vi "PD4-C Setup State Machine.vi"(11 "Boolean in":refnum<vi>) -> (0 "error out":errorcluster, 2 "Answer":i32, 3 "VISA Refnum out":refnum<visa-resource-name>)   [LabVIEW 2021]
uses:
  Nanotech PDC-4.lvlib
  <vilib>/Utility/error.llb/Error Cluster From Error Code.vi
  <vilib>/ErrorRing/Error Ring.xnode
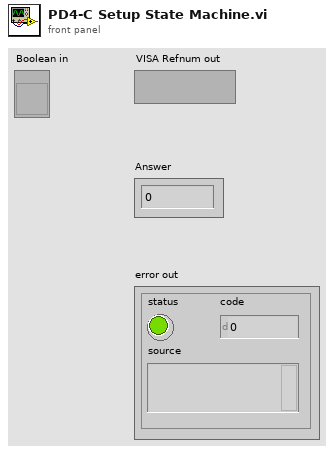
[diagram p1: front panel]
types:
  T1 = cluster{"Data (dec)":i32, "write":bool, "Index":string, "Sub-Index":string, "Data-Size (in Byte)":u8}
  T2 = cluster{"Index":string, "Sub-Index":string, "Data-Size (in Byte)":u8}
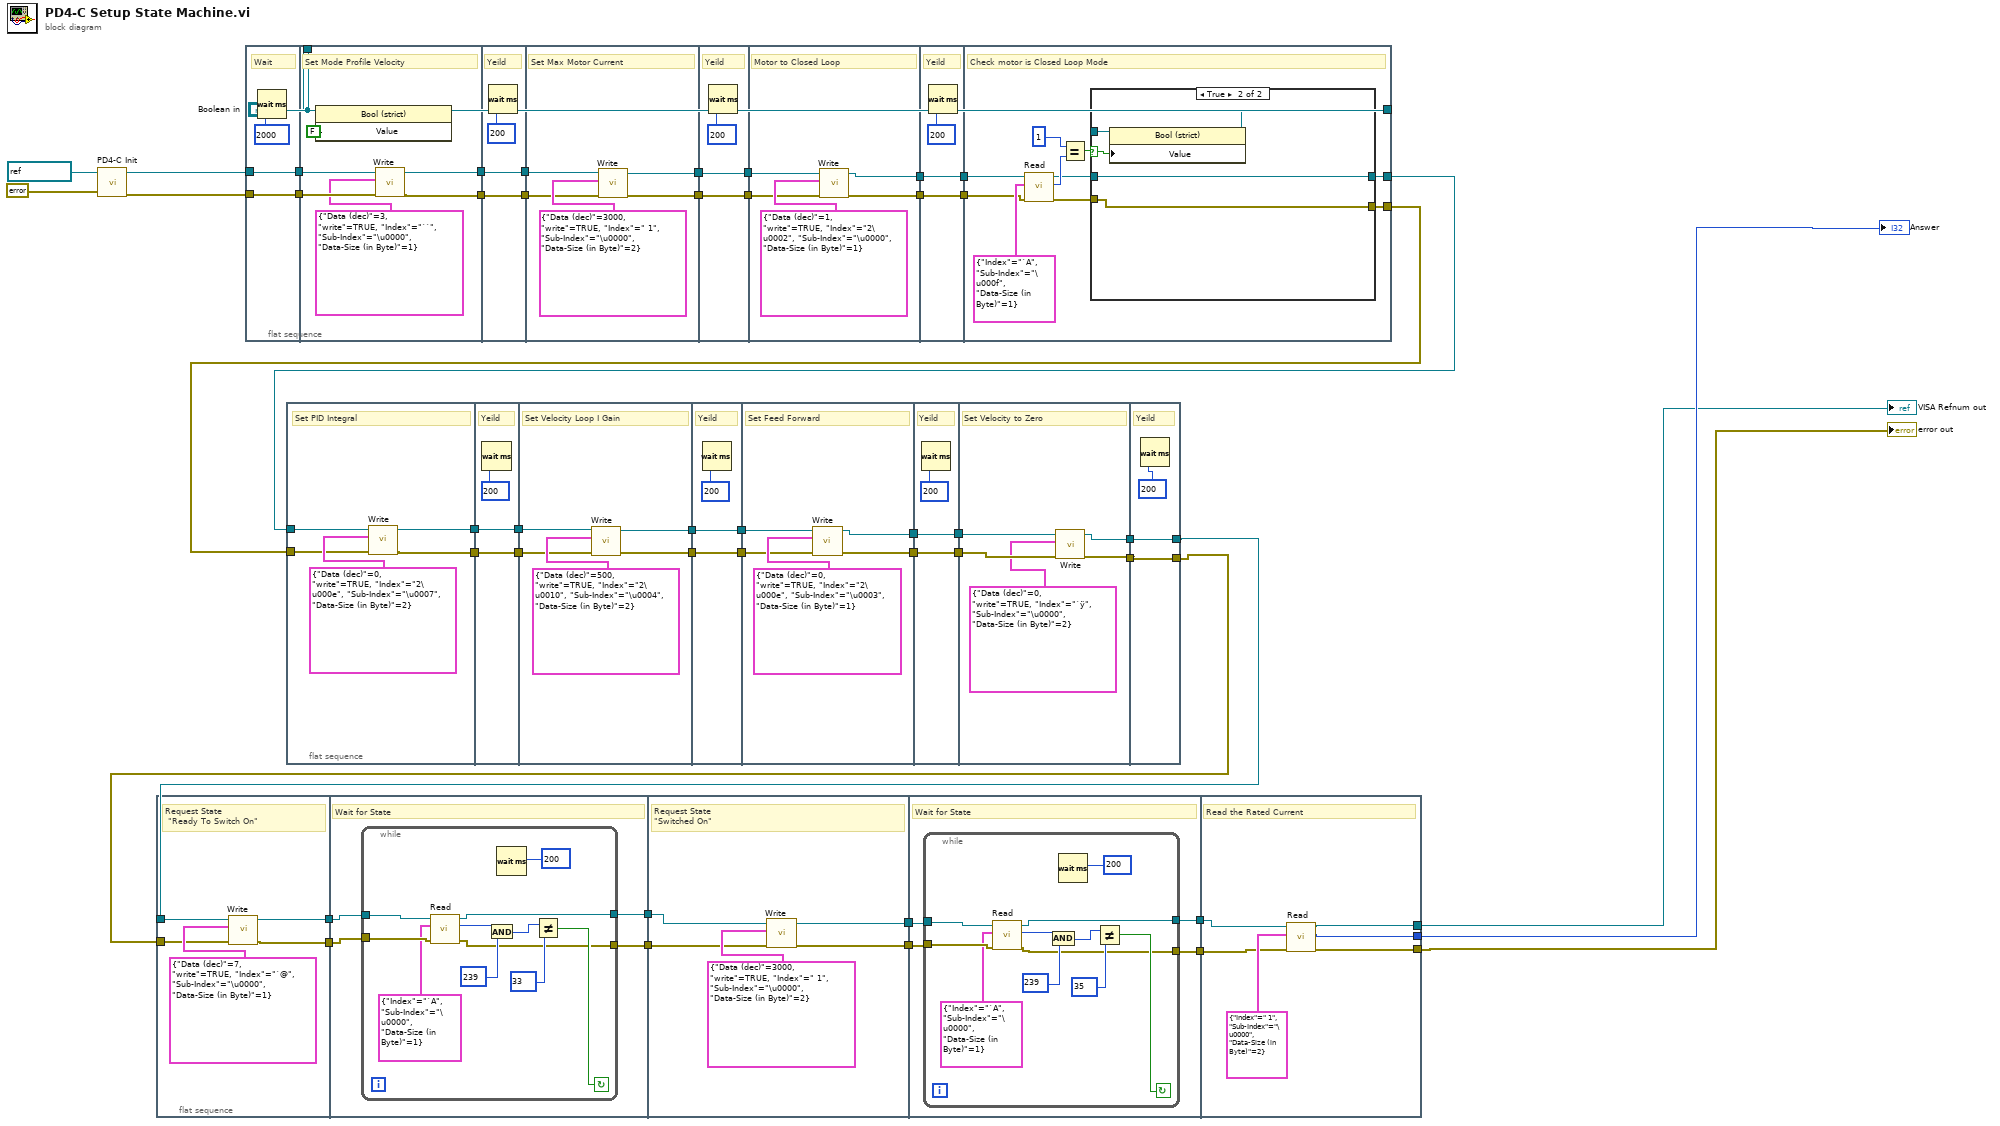
[diagram p0: block diagram]
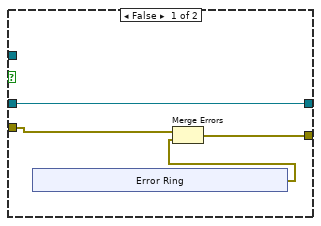
[diagram p2: hidden frame]
diagram:
  n1 = call "PD4-C Init.vi"("error in (no error)"=errorcluster {"status"=FALSE, "code"=0, "source"=""}, "VISA Refnum in"=refnum<visa-resource-name> "COM15") -> ("error out"=w4:errorcluster, "VISA Refnum out"=w5:refnum<visa-resource-name>)  [unwired: 8 in]
  n2 = flat-sequence {
    tunnel: [w52] -> w20
    tunnel: [w51] -> w19
    tunnel: w8 -> [w50]
    tunnel: w9 -> [w49]
    tunnel: w20 -> [w56]
    tunnel: w19 -> [w57]
    tunnel: [w55] -> w18
    tunnel: [w54] -> w17
    tunnel: [w72] -> w16
    tunnel: [w71] -> w15
    tunnel: w18 -> [w70]
    tunnel: w17 -> [w69]
    tunnel: w16 -> [w76]
    tunnel: w15 -> [w77]
    tunnel: [w75] -> w14
    tunnel: [w74] -> w13
    tunnel: w14 -> [w92]
    tunnel: w13 -> [w93]
    tunnel: [w91] -> w10
    tunnel: [w90] -> w11
    tunnel: [w89] -> w12
    frame #0 {
      # "Request State\n \"Ready To Switch On\""
      n3 = call "Write.vi"("error in"=w49, "Write"=T1 {"Data (dec)"=7, "write"=TRUE, "Index"="`@", "Sub-Index"="\u0000", "Data-Size (in Byte)"=1}, "ComPort In"=w50) -> ("error out"=w52:errorcluster, "ComPort Out"=w51:refnum<visa-resource-name>)  [unwired: 7 in]
    }
    frame #1 {
      # "Wait for State"
      n4 = while {
        tunnel: w57 -> [w67]
        tunnel: w56 -> [w66]
        tunnel: [w59] -> w55
        tunnel: [w58] -> w54
        stop <- w60 continue-if-true
        n5 = call "Read.vi"("error out"=w66, "Command"=T2 {"Index"="`A", "Sub-Index"="\u0000", "Data-Size (in Byte)"=1}, "ComPort In"=w67) -> ("error out 2"=w58:errorcluster, "Answer"=w64:i32, "ComPort Out"=w59:refnum<visa-resource-name>)  [unwired: 6 in]
        n6 = And(x=w64, y=239) -> (x .and. y?=w62:i32)
        n7 = Wait (ms)(milliseconds to wait=u32 200) -> ()  [unwired: 1 out]
        n8 = Not Equal?(x=w62, y=33) -> (x != y?=w60:bool)
      }
    }
    frame #2 {
      # "Request State\n\"Switched On\""
      n9 = call "Write.vi"("error in"=w69, "Write"=T1 {"Data (dec)"=3000, "write"=TRUE, "Index"=" 1", "Sub-Index"="\u0000", "Data-Size (in Byte)"=2}, "ComPort In"=w70) -> ("error out"=w71:errorcluster, "ComPort Out"=w72:refnum<visa-resource-name>)  [unwired: 7 in]
    }
    frame #3 {
      # "Wait for State"
      n10 = while {
        tunnel: w76 -> [w87]
        tunnel: w77 -> [w86]
        tunnel: [w79] -> w75
        tunnel: [w78] -> w74
        stop <- w80 continue-if-true
        n11 = call "Read.vi"("error out"=w86, "Command"=T2 {"Index"="`A", "Sub-Index"="\u0000", "Data-Size (in Byte)"=1}, "ComPort In"=w87) -> ("error out 2"=w78:errorcluster, "Answer"=w84:i32, "ComPort Out"=w79:refnum<visa-resource-name>)  [unwired: 6 in]
        n12 = And(x=w84, y=239) -> (x .and. y?=w82:i32)
        n13 = Wait (ms)(milliseconds to wait=u32 200) -> ()  [unwired: 1 out]
        n14 = Not Equal?(x=w82, y=35) -> (x != y?=w80:bool)
      }
    }
    frame #4 {
      # "Read the Rated Current"
      n15 = call "Read.vi"("error out"=w93, "Command"=T2 {"Index"=" 1", "Sub-Index"="\u0000", "Data-Size (in Byte)"=2}, "ComPort In"=w92) -> ("error out 2"=w90:errorcluster, "Answer"=w89:i32, "ComPort Out"=w91:refnum<visa-resource-name>)  [unwired: 6 in]
    }
  }
  n16 = flat-sequence {
    tunnel: [w96] -> w48
    tunnel: w4 -> [w96]
    tunnel: [w95] -> w47
    tunnel: w5 -> [w95]
    tunnel: w48 -> [w104]
    tunnel: w47 -> [w103]
    tunnel: [w101] -> w46
    tunnel: [w100] -> w45
    tunnel: "Boolean in" -> [w98]
    tunnel: [w106] -> w44
    tunnel: w46 -> [w106]
    tunnel: [w105] -> w43
    tunnel: w45 -> [w105]
    tunnel: w44 -> [w111]
    tunnel: w43 -> [w110]
    tunnel: [w109] -> w42
    tunnel: [w108] -> w41
    tunnel: [w114] -> w40
    tunnel: w42 -> [w114]
    tunnel: [w113] -> w39
    tunnel: w41 -> [w113]
    tunnel: w40 -> [w119]
    tunnel: w39 -> [w118]
    tunnel: [w117] -> w38
    tunnel: [w116] -> w37
    tunnel: w38 -> [w122]
    tunnel: [w122] -> w36
    tunnel: [w121] -> w35
    tunnel: w37 -> [w121]
    tunnel: w36 -> [w133]
    tunnel: w35 -> [w132]
    tunnel: [w127] -> w6
    tunnel: [w125] -> w7
    tunnel: "Boolean in" -> [w124]
    frame #0 {
      # "Wait"
      n17 = Wait (ms)(milliseconds to wait=u32 2000) -> ()  [unwired: 1 out]
    }
    frame #1 {
      # "Set Mode Profile Velocity"
      n18 = property on="Property Node" class="Bool (strict)"(reference=w98, "Value"=FALSE ("Closed Loop Available")) -> ()  [unwired: 1 in, 2 out]
      n19 = call "Write.vi"("error in"=w104, "Write"=T1 {"Data (dec)"=3, "write"=TRUE, "Index"="``", "Sub-Index"="\u0000", "Data-Size (in Byte)"=1}, "ComPort In"=w103) -> ("error out"=w101:errorcluster, "ComPort Out"=w100:refnum<visa-resource-name>)  [unwired: 7 in]
    }
    frame #2 {
      # "Yeild"
      n20 = Wait (ms)(milliseconds to wait=u32 200) -> ()  [unwired: 1 out]
    }
    frame #3 {
      # "Set Max Motor Current"
      n21 = call "Write.vi"("error in"=w111, "Write"=T1 {"Data (dec)"=3000, "write"=TRUE, "Index"=" 1", "Sub-Index"="\u0000", "Data-Size (in Byte)"=2}, "ComPort In"=w110) -> ("error out"=w108:errorcluster, "ComPort Out"=w109:refnum<visa-resource-name>)  [unwired: 7 in]
    }
    frame #4 {
      # "Yeild"
      n22 = Wait (ms)(milliseconds to wait=u32 200) -> ()  [unwired: 1 out]
    }
    frame #5 {
      # "Motor to Closed Loop"
      n23 = call "Write.vi"("error in"=w118, "Write"=T1 {"Data (dec)"=1, "write"=TRUE, "Index"="2\u0002", "Sub-Index"="\u0000", "Data-Size (in Byte)"=1}, "ComPort In"=w119) -> ("error out"=w117:errorcluster, "ComPort Out"=w116:refnum<visa-resource-name>)  [unwired: 7 in]
    }
    frame #6 {
      # "Yeild"
      n24 = Wait (ms)(milliseconds to wait=u32 200) -> ()  [unwired: 1 out]
    }
    frame #7 {
      # "Check motor is Closed Loop Mode"
      n25 = call "Read.vi"("error out"=w133, "Command"=T2 {"Index"="`A", "Sub-Index"="\u000f", "Data-Size (in Byte)"=1}, "ComPort In"=w132) -> ("error out 2"=w126:errorcluster, "Answer"=w131:i32, "ComPort Out"=w128:refnum<visa-resource-name>)  [unwired: 6 in]
      n26 = Equal?(x=1, y=w131) -> (x = y?=w129:bool)
      n27 = case shown="True" w129 {
        selector: w129 -> [_ w147]
        tunnel: [w138 w146] -> w127
        tunnel: w128 -> [w138 w146]
        tunnel: w126 -> [w137 w145]
        tunnel: [w135 w145] -> w125
        tunnel: w124 -> [_ w144]
        frame False {
          n28 = xnode "Error Ring"() -> ("error out"=w136:errorcluster)
          n29 = Merge Errors(w137, w136) -> (w135:errorcluster)
        }
        frame True {
          n30 = property on="Property Node" class="Bool (strict)"(reference=w144, "Value"=w147) -> ()  [unwired: 1 in, 2 out]
        }
      }
    }
  }
  n31 = flat-sequence {
    tunnel: [w151] -> w34
    tunnel: [w150] -> w33
    tunnel: w6 -> [w149]
    tunnel: w7 -> [w148]
    tunnel: [w154] -> w32
    tunnel: w34 -> [w154]
    tunnel: [w153] -> w31
    tunnel: w33 -> [w153]
    tunnel: w32 -> [w159]
    tunnel: w31 -> [w158]
    tunnel: [w157] -> w30
    tunnel: [w156] -> w29
    tunnel: [w162] -> w28
    tunnel: w30 -> [w162]
    tunnel: [w161] -> w27
    tunnel: w29 -> [w161]
    tunnel: w28 -> [w167]
    tunnel: w27 -> [w166]
    tunnel: [w165] -> w26
    tunnel: [w164] -> w25
    tunnel: w26 -> [w170]
    tunnel: [w170] -> w24
    tunnel: [w169] -> w23
    tunnel: w25 -> [w169]
    tunnel: w24 -> [w175]
    tunnel: w23 -> [w176]
    tunnel: [w174] -> w22
    tunnel: [w173] -> w21
    tunnel: [w178] -> w9
    tunnel: w22 -> [w178]
    tunnel: w21 -> [w177]
    tunnel: [w177] -> w8
    frame #0 {
      # "Set PID Integral"
      n32 = call "Write.vi"("error in"=w148, "Write"=T1 {"Data (dec)"=0, "write"=TRUE, "Index"="2\u000e", "Sub-Index"="\u0007", "Data-Size (in Byte)"=2}, "ComPort In"=w149) -> ("error out"=w151:errorcluster, "ComPort Out"=w150:refnum<visa-resource-name>)  [unwired: 7 in]
    }
    frame #1 {
      # "Yeild"
      n33 = Wait (ms)(milliseconds to wait=u32 200) -> ()  [unwired: 1 out]
    }
    frame #2 {
      # "Set Velocity Loop I Gain"
      n34 = call "Write.vi"("error in"=w159, "Write"=T1 {"Data (dec)"=500, "write"=TRUE, "Index"="2\u0010", "Sub-Index"="\u0004", "Data-Size (in Byte)"=2}, "ComPort In"=w158) -> ("error out"=w156:errorcluster, "ComPort Out"=w157:refnum<visa-resource-name>)  [unwired: 7 in]
    }
    frame #3 {
      # "Yeild"
      n35 = Wait (ms)(milliseconds to wait=u32 200) -> ()  [unwired: 1 out]
    }
    frame #4 {
      # "Set Feed Forward"
      n36 = call "Write.vi"("error in"=w166, "Write"=T1 {"Data (dec)"=0, "write"=TRUE, "Index"="2\u000e", "Sub-Index"="\u0003", "Data-Size (in Byte)"=1}, "ComPort In"=w167) -> ("error out"=w165:errorcluster, "ComPort Out"=w164:refnum<visa-resource-name>)  [unwired: 7 in]
    }
    frame #5 {
      # "Yeild"
      n37 = Wait (ms)(milliseconds to wait=u32 200) -> ()  [unwired: 1 out]
    }
    frame #6 {
      # "Set Velocity to Zero"
      n38 = call "Write.vi"("error in"=w175, "Write"=T1 {"Data (dec)"=0, "write"=TRUE, "Index"="`ÿ", "Sub-Index"="\u0000", "Data-Size (in Byte)"=2}, "ComPort In"=w176) -> ("error out"=w174:errorcluster, "ComPort Out"=w173:refnum<visa-resource-name>)  [unwired: 7 in]
    }
    frame #7 {
      # "Yeild"
      n39 = Wait (ms)(milliseconds to wait=u32 200) -> ()  [unwired: 1 out]
    }
  }
  "Answer" <- w12
  "error out" <- w11
  "VISA Refnum out" <- w10
